vi "RGB Image to GrayScale.vi"(6 "error in (no error)":errorcluster, 9 "path to BMP file":path) -> (0 "error out":errorcluster, 3 "RGB GrayScale":picture)   [LabVIEW 2016]
uses:
  <vilib>/picture/picture.llb/Draw True-Color Pixmap.vi
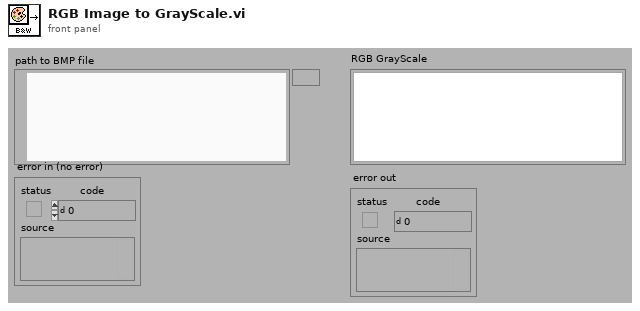
[diagram p1: front panel]
types:
  T1 = typedef "imagedata.ctl" = cluster{"image type":i32, "image depth":i32, "image":u8[], "mask":u8[], "colors":u32[], "Rectangle":cluster{"left":i16, "top":i16, "right":i16, "bottom":i16}}
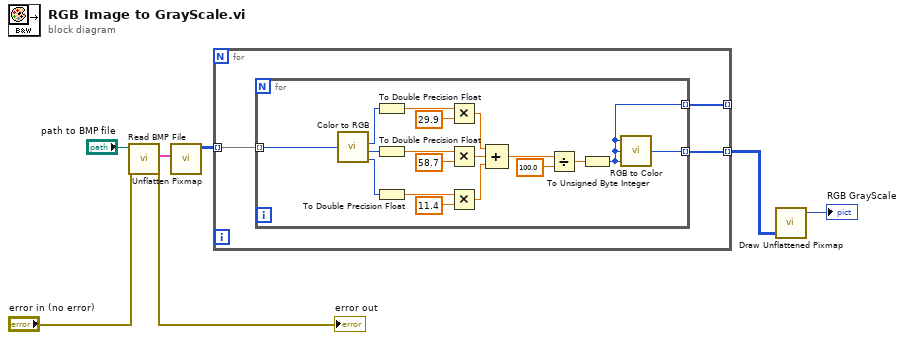
[diagram p0: block diagram]
diagram:
  n1 = call <vilib>:"Read BMP File.vi"("error in (no error)"="error in (no error)", "path to BMP file"="path to BMP file") -> ("error out"=→"error out":errorcluster, "image data"=w4:T1)  [unwired: 7 in, 1 out]
  n2 = call <vilib>:"Unflatten Pixmap.vi"("image data"=w4) -> ("24-bit pixmap"=w5:u32[][])  [unwired: 4 in, 6 out]
  n3 = for {
    tunnel: w5 -> [w10] mode=indexing
    tunnel: [w9] -> _ mode=indexing
    tunnel: [w8] -> w3 mode=indexing
    n4 = for {
      tunnel: w10 -> [w28] mode=indexing
      tunnel: [w11] -> w9 mode=indexing
      tunnel: [w12] -> w8 mode=indexing
      n5 = call <vilib>:"Color to RGB.vi"("Color"=w28) -> ("R"=w27:u8, "G"=w25:u8, "B"=w24:u8)  [unwired: 1 out]
      n6 = To Double Precision Float(number=w27) -> (double precision float=w26:dbl)
      n7 = To Double Precision Float(number=w25) -> (double precision float=w23:dbl)
      n8 = To Double Precision Float(number=w24) -> (double precision float=w22:dbl)
      n9 = Multiply(x=w26, y=29.9) -> (x*y=w18:dbl)
      n10 = Multiply(x=w23, y=58.7) -> (x*y=w17:dbl)
      n11 = Multiply(x=w22, y=11.4) -> (x*y=w16:dbl)
      n12 = Compound Arithmetic op=ADD(w18, w17, w16) -> (w15:dbl)
      n13 = Divide(x=w15, y=100.0) -> (x/y=w13:dbl)
      n14 = To Unsigned Byte Integer(number=w13) -> (unsigned 8bit integer=w11:u8)
      n15 = call <vilib>:"RGB to Color.vi"("B"=w11, "G"=w11, "R"=w11) -> ("Color"=w12:u32)
    }
  }
  n16 = call-poly <vilib>:"Draw Unflattened Pixmap.vi"("data (RGB format)"=w3) -> ("new picture"=→"RGB GrayScale":picture)  [unwired: 8 in]
